vi "Evaluate Part 1.vi"() -> ()   [LabVIEW 2021]
uses:
  Proto/Maze.lvclass
  Beam/Beam.lvclass
panel:
  out "size(s)":i32
  in  "Input":string=".|...\\....\n|.-.\\.....\n.....|-...\n........|.\n..........\n.........\\\n..../.\\\\..\n.-.-/..|..\n.|....-|.\\\n..//.|...."
  # "6883"
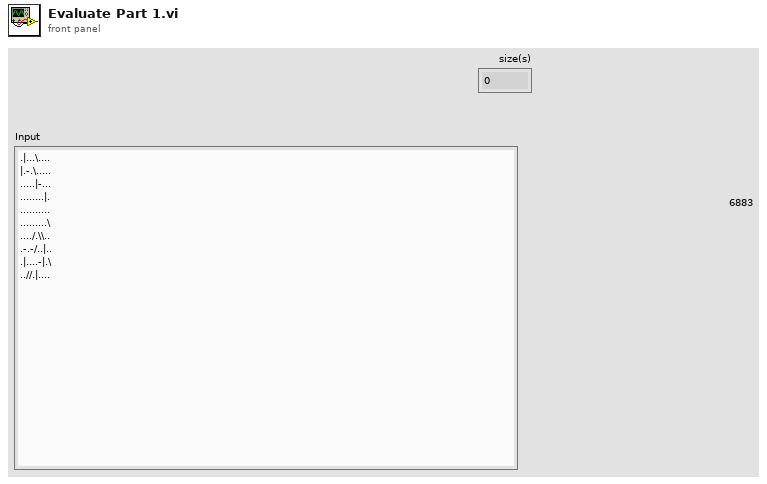
[diagram p1: front panel]
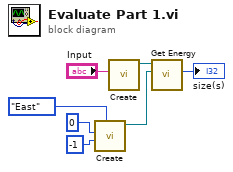
[diagram p0: block diagram]
diagram:
  n1 = call "Create.vi"("Direction"=enum16{"North", "East", "South", "West"}."East", "Col"=-1, "Row"=0) -> ("Beam"=w2:refnum<class "Beam.lvclass">)  [unwired: 7 in, 1 out]
  n2 = call "Create.vi"("Input"="Input") -> ("Proto"=w3:refnum<class "Maze.lvclass">)  [unwired: 7 in, 3 out]
  n3 = call "Get Energy.vi"("Beam"=w2, "Maze in"=w3) -> ("Numeric"=→"size(s)":i32)  [unwired: 9 in]
